vi "WorkingWithArrays1.vi"() -> ()   [LabVIEW 2014]
panel:
  out "Modified Array":dbl[](array[numeric])
  out "Output":dbl
  in  "index":i32
  in  "Array":dbl[](array[numeric])
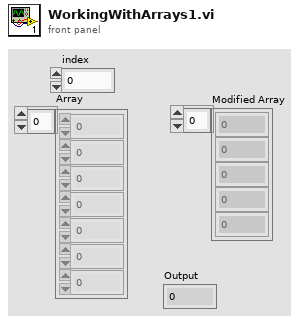
[diagram p1: front panel]
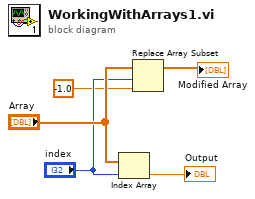
[diagram p0: block diagram]
diagram:
  n1 = Index Array(array="Array", index="index") -> (element=→"Output":dbl)
  n2 = Replace Array Subset(array="Array", new element=-1.0 ("new element/subarray"), index="index") -> (→"Modified Array":dbl[])
